vi "[FGV] Analysis_Result_Points.vi"(6 "CoordSystemRun":bool=TRUE, 7 "Action":T2, 8 "error in (no error)":errorcluster, 10 "Analysis_Point_Result":T1[](array[typedef])) -> (0 "error out":errorcluster, 2 "Analysis_Point_Result Out":T1[](array[typedef]))   [LabVIEW 2019]
uses:
  Controls/AnalysisResultPointsAction.ctl
  Analysis/Controls/Analysis_Result_To_Caliper.ctl
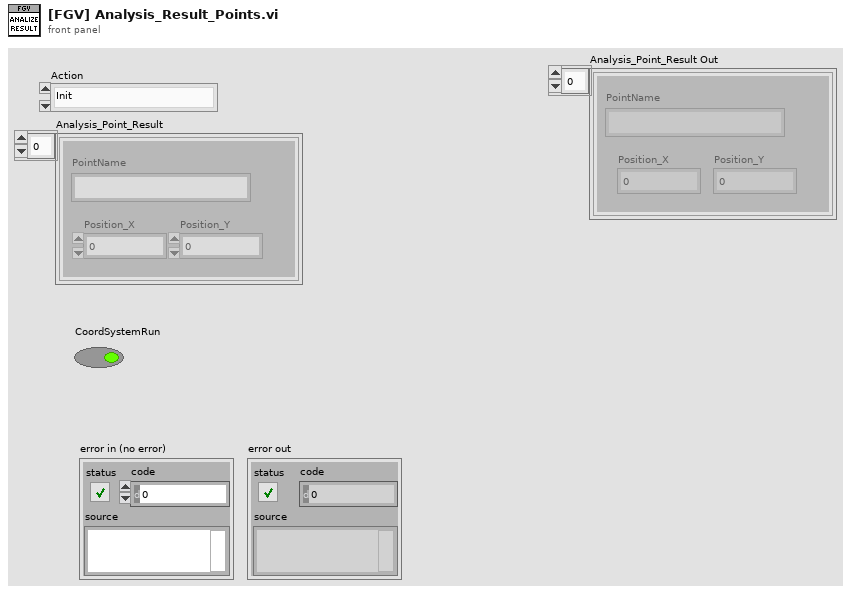
[diagram p1: front panel]
types:
  T1 = typedef "Analysis_Result_To_Caliper.ctl" = cluster{"PointName":string, "Position_X":dbl, "Position_Y":dbl}
  T2 = typedef "AnalysisResultPointsAction.ctl" = enum16{"Init", "Add", "Delete", "ReplaceAll", "ReadAll", "Close"}
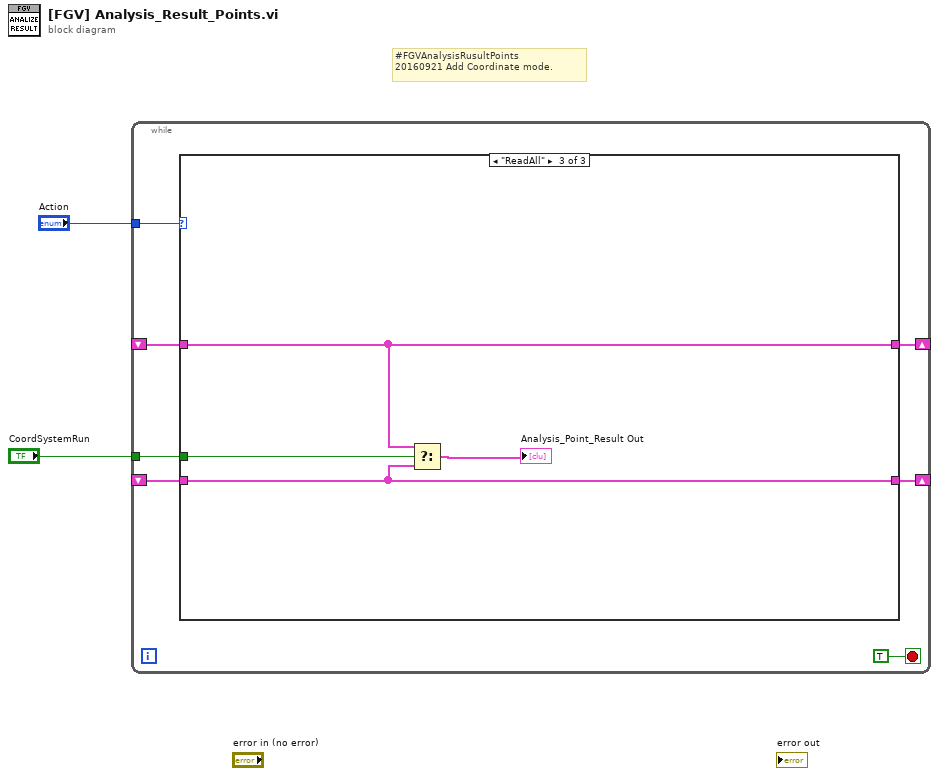
[diagram p0: block diagram]
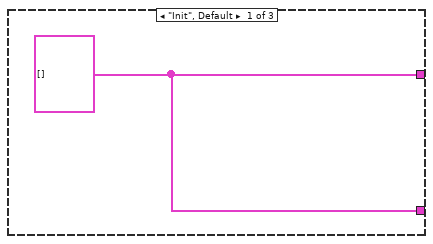
[diagram p2: hidden frame]
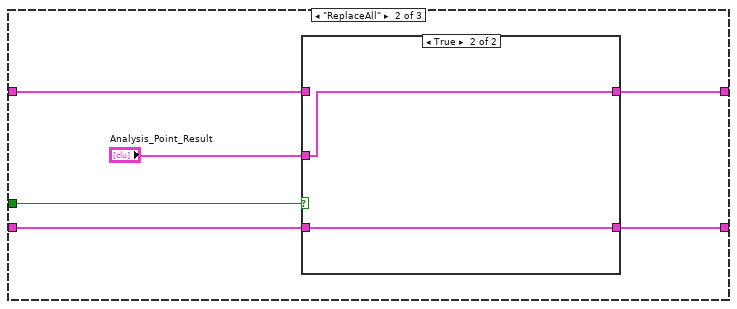
[diagram p3: hidden frame]
diagram:
  # "#FGVAnalysisRusultPoints\n20160921 Add Coordinate mode."
  n1 = while {
    tunnel: "Action" -> [w8]
    shift-right: [w7] -> _
    shift-left: _ -> [w6]
    shift-right: [w5] -> _
    shift-left: _ -> [w4]
    tunnel: "CoordSystemRun" -> [w3]
    stop <- TRUE stop-if-true
    n2 = case shown="\"ReadAll\"" w8 {
      tunnel: [w10 w15 w23] -> w7
      tunnel: w6 -> [_ w14 w23]
      tunnel: [w10 w13 w22] -> w5
      tunnel: w4 -> [_ w12 w22]
      tunnel: w3 -> [_ w11 w24]
      frame "Init", Default {
        w10 = T1[] [] ("Analysis_Point_Result")
      }
      frame "ReplaceAll" {
        n3 = case shown="True" w11 {
          tunnel: "Analysis_Point_Result" -> [w17 w20]
          tunnel: [w18 w20] -> w15
          tunnel: w14 -> [w18 _]
          tunnel: [w17 w19] -> w13
          tunnel: w12 -> [_ w19]
          frame False {
          }
          frame True {
          }
        }
      }
      frame "ReadAll" {
        n4 = Select(t=w23, s=w24, f=w22) -> (s? t:f=→"Analysis_Point_Result Out":T1[])
      }
    }
  }
